vi "stage_toggle.vi"(8 "error in (no error)":errorcluster, 9 "Engage?":bool, 10 "Stage Name":string, 11 "newport_xps in":refnum<class "newport_xps.lvclass">) -> (0 "error out":errorcluster, 3 "newport_xps out":refnum<class "newport_xps.lvclass">)   [LabVIEW 2015, in "newport_xps.lvclass"]
uses:
  newport_xps.lvclass
  newport_xps.lvclass/newport_xps.ctl
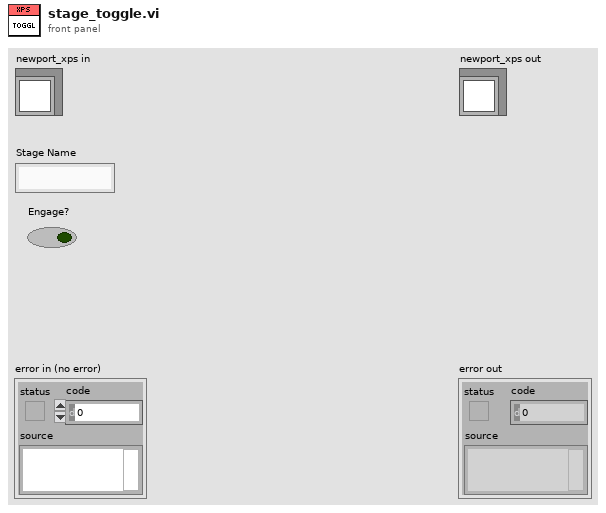
[diagram p1: front panel]
types:
  T1 = cluster{"connection TCP":refnum<k5>, "LogTo File":bool, "Log File refnum":refnum<file>, "no error if error log":bool}
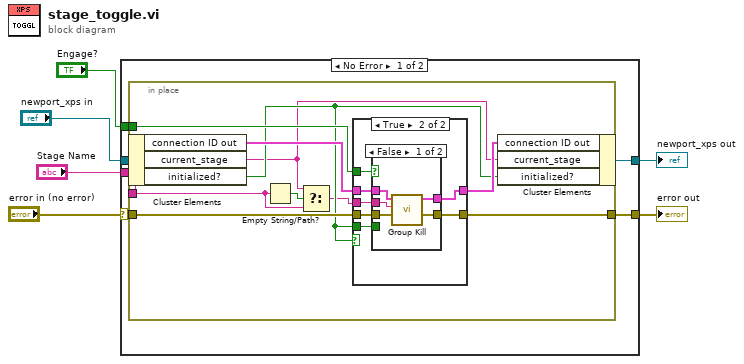
[diagram p0: block diagram]
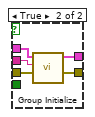
[diagram p3: hidden frame]
diagram:
  n1 = case shown="No Error" "error in (no error)" {
    selector: "error in (no error)" -> [w9 w42]
    tunnel: "newport_xps in" -> [w12 w43]
    tunnel: [w11 w43] -> w4
    tunnel: "Engage?" -> [w10 _]
    tunnel: [w8 w42] -> w2
    tunnel: "Stage Name" -> [w7 _]
    frame No Error {
      n2 = in-place {
        in-place-border: w10 -> [w18]
        in-place-border: w9 -> [w20]
        in-place-border: [w19] -> w8
        in-place-border: w7 -> [w15]
        n3 = in-place-cluster #1(w12) -> ("connection ID out"=w22:T1, "current_stage"=w14:string, "initialized?"=w17:bool)
        n4 = Empty String/Path?(string/path=w15) -> (empty?=w16:bool)
        n5 = Select(t=w14, s=w16, f=w15) -> (s? t:f=w13:string)
        n6 = case shown="True" w17 {
          tunnel: w22 -> [w24 w31]
          tunnel: [w24 w30] -> w21
          tunnel: w13 -> [_ w29]
          tunnel: w20 -> [w23 w28]
          tunnel: [w23 w27] -> w19
          tunnel: w18 -> [_ w26]
          tunnel: w17 -> [_ w25]
          frame False {
          }
          frame True {
            n7 = case shown="False" w26 {
              tunnel: w31 -> [w36 w41]
              tunnel: [w35 w40] -> w30
              tunnel: w29 -> [w34 w39]
              tunnel: w28 -> [w33 w38]
              tunnel: [w32 w37] -> w27
              tunnel: w25 -> [_ _]
              frame False {
                n8 = call "Group Kill.vi"("XPS error in (no error)"=w33, "Group Name (250 c max)"=w34, "connection ID in"=w36) -> ("XPS error out"=w32:errorcluster, "connection ID out"=w35:T1)  [unwired: 6 in, 1 out]
              }
              frame True {
                n9 = call "Group Initialize.vi"("XPS error in (no error)"=w38, "Group Name (250 c max)"=w39, "connection ID in"=w41) -> ("XPS error out"=w37:errorcluster, "connection ID out"=w40:T1)  [unwired: 6 in, 1 out]
              }
            }
          }
        }
        n10 = in-place-cluster #1("connection ID out"=w21, "current_stage"=w14, "initialized?"=w17) -> (w11:refnum<class "newport_xps.lvclass">)
      }
    }
    frame Error {
    }
  }
  "error out" <- w2
  "newport_xps out" <- w4
